vi "PythonNode_AddTwoIntegers.vi"() -> ()   [LabVIEW 2021]
doc: "This example demonstrates how to call a Python function and pass integers as arguments. It uses a python function to compute the sum of two integers."
panel:
  out "Array":i32[](array[numeric])
  out "error out":errorcluster
  in  "aantal frames":i32=41
  in  "error in (no error)":errorcluster
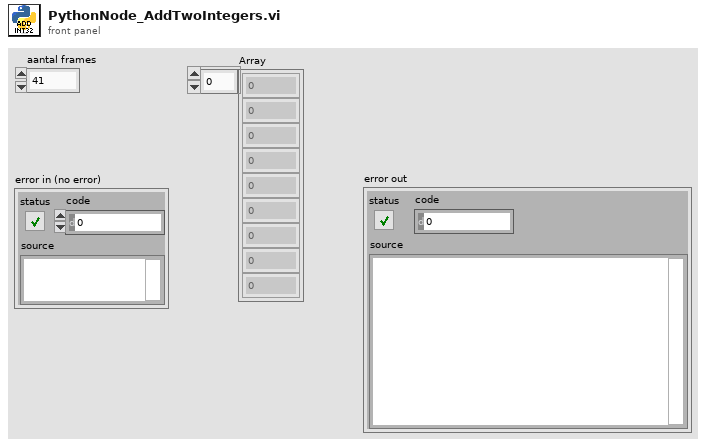
[diagram p1: front panel]
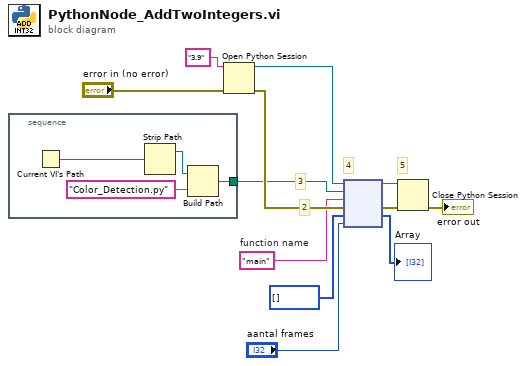
[diagram p0: block diagram]
diagram:
  w8 = "main"  # function name
  # "5"
  # "4"
  # "2"
  # "3"
  n1 = stacked-sequence {
    tunnel: [w16] -> w9
    frame #0 {
      n2 = Current VI's Path() -> (path=w13:path)
      n3 = Strip Path(path=w13) -> (stripped path=w14:path)  [unwired: 1 out]
      n4 = Build Path(base path=w14, name or relative path="Color_Detection.py") -> (appended path=w16:path)
    }
  }
  n5 = Open Python Session(python version="3.9", 3:"error in (no error)") -> (session out=w11:refnum<k35>, error out=w10:errorcluster)  [unwired: 1 in]
  n6 = node(w11, w9, w8, w10, i32[] [], "aantal frames") -> (w7:refnum<k35>, w6:errorcluster, →"Array":i32[])  [unwired: 1 in, 2 out]
  n7 = Close Python Session(session in=w7, error in=w6) -> (11:→"error out":errorcluster)
